vi "Read ini.vi"(8 "error in (no error)":errorcluster, 11 "Sett data":T1={"Filter"=0, "Gain"=0.0, "Bit rate"=0.0, "ISO/IEC w "=enum."14443 Type A", "BI"={"R"=0.0, "C"=0.0, "L"=0.0}, "BM"={"R"=0.0, "C"=0.0, "L"=0.0}, "M"={"Метка"=4, "Считыветель"=4}, "Type noise"=enum."Гауссовский шум", "Link"=enum."UPLINK", "Noise attenuator"=0.0, "Signal gain"=1.0, "Distance"=0.0} {"Distance" scale=0.0..10.0; "Signal gain" min=1.0 max=100.0 step=1.0 scale=1.0..30.0; "Noise attenuator" scale=0.01..1.01; "M"."Считыветель" min=4 max=128 step=4; "M"."Метка" min=4 max=128 step=4; "Bit rate" min=4.0 max=128.0 step=4.0}) -> (0 "error out":errorcluster, 3 "Sett data out":T1={"Filter"=0, "Gain"=0.0, "Bit rate"=0.0, "ISO/IEC w "=enum."14443 Type A", "BI"={"R"=0.0, "C"=0.0, "L"=0.0}, "BM"={"R"=0.0, "C"=0.0, "L"=0.0}, "M"={"Метка"=4, "Считыветель"=4}, "Type noise"=enum."Гауссовский шум", "Link"=enum."UPLINK", "Noise attenuator"=0.0, "Signal gain"=1.0, "Distance"=0.0} {"Distance" scale=0.0..10.0; "Signal gain" min=1.0 max=100.0 step=1.0 scale=1.0..30.0; "Noise attenuator" scale=0.01..1.01; "M"."Считыветель" min=4 max=128 step=4; "M"."Метка" min=4 max=128 step=4; "Bit rate" min=4.0 max=128.0 step=4.0})   [LabVIEW 2019]
uses:
  TypeDef/Sett data.ctl
  TypeDef/ISO.ctl
  TypeDef/Noise.ctl
  TypeDef/Link.ctl
  <vilib>/Utility/config.llb/Read Key (I32).vi
  <vilib>/Utility/config.llb/Read Key (Double).vi
  <vilib>/Utility/config.llb/NI_LVConfig.lvlib
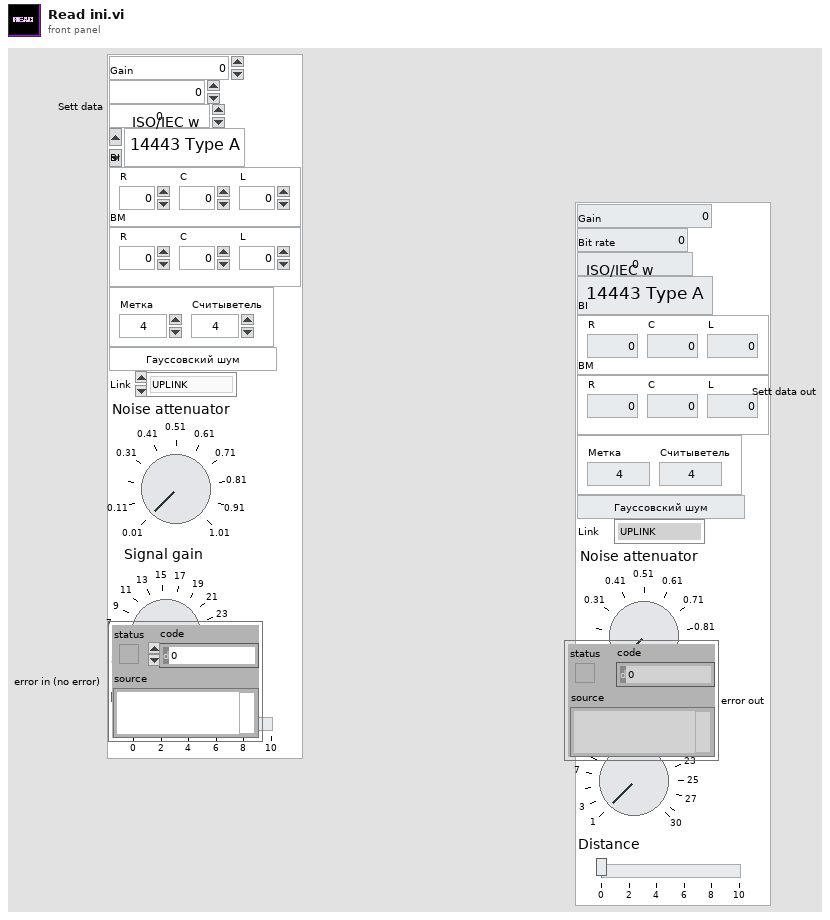
[diagram p1: front panel]
types:
  T1 = typedef "Sett data.ctl" = cluster{"Filter":i32, "Gain":dbl, "Bit rate":dbl, "ISO/IEC w ":T2, "BI":cluster{"R":dbl, "C":dbl, "L":dbl}, "BM":cluster{"R":dbl, "C":dbl, "L":dbl}, "M":cluster{"Метка":i64, "Считыветель":i64}, "Type noise":T3, "Link":T4, "Noise attenuator":dbl, "Signal gain":dbl, "Distance":dbl}
  T2 = typedef "ISO.ctl" = enum16{"14443 Type A", "14443 Type B", "Felica", "15693"}
  T3 = typedef "Noise.ctl" = enum16{"Гауссовский шум", "Белый шум"}
  T4 = typedef "Link.ctl" = enum16{"UPLINK", "DOWNLINK"}
  T5 = typedef "NI_LVConfig.lvlib/Config Data RefNum.ctl" = refnum<k1>
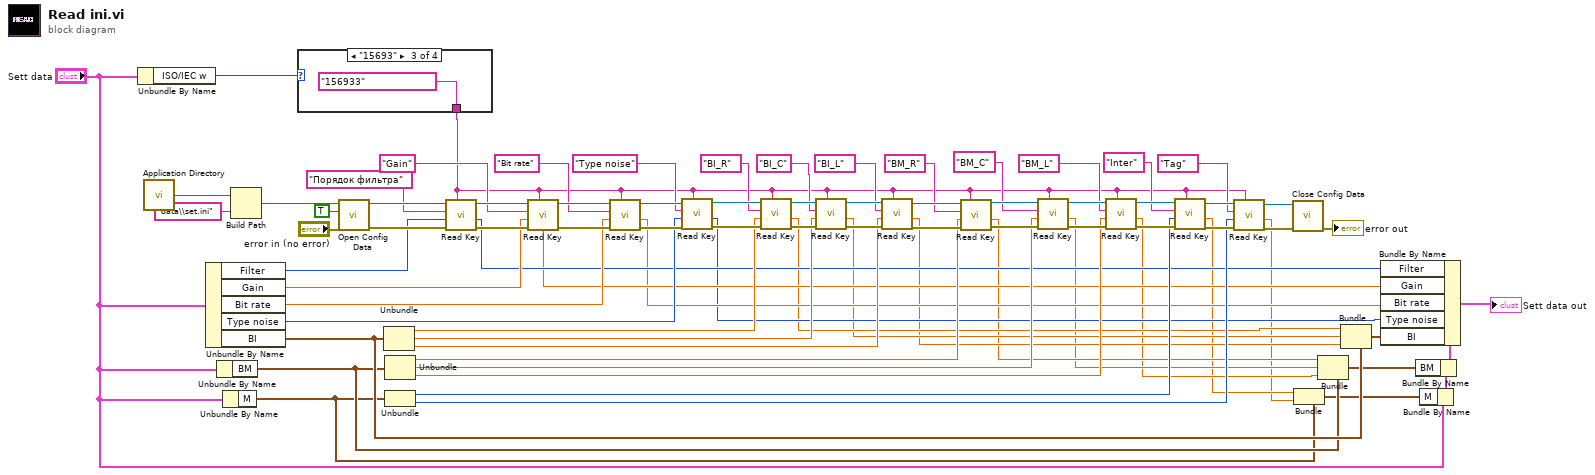
[diagram p0: block diagram]
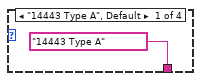
[diagram p2: hidden frame]
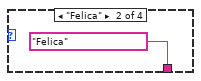
[diagram p3: hidden frame]
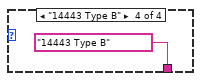
[diagram p4: hidden frame]
diagram:
  n1 = Unbundle By Name("Sett data") -> ("ISO/IEC w"=w73:T2)
  n2 = call <vilib>:"Application Directory.vi"() -> ("Application Directory"=w80:path)
  n3 = Unbundle By Name("Sett data") -> ("Filter"=w62:i32, "Gain"=w59:dbl, "Bit rate"=w58:dbl, "Type noise"=w56:T3, "BI"=w15:cluster{"R":dbl, "C":dbl, "L":dbl})
  n4 = Unbundle By Name("Sett data") -> ("BM"=w10:cluster{"R":dbl, "C":dbl, "L":dbl})
  n5 = Unbundle By Name("Sett data") -> ("M"=w4:cluster{"Метка":i64, "Считыветель":i64})
  n6 = Build Path(base path=w80, name or relative path="data\\set.ini") -> (appended path=w78:path)
  n7 = case shown="\"15693\"" w73 {
    tunnel: ["14443 Type A" "Felica" "156933" "14443 Type B"] -> w23
    frame "14443 Type A", Default {
    }
    frame "Felica" {
    }
    frame "15693" {
    }
    frame "14443 Type B" {
    }
  }
  n8 = call <vilib>:"Open Config Data.vi"("error in (no error)"="error in (no error)", "create file if necessary (T)"=TRUE, "configuration file path"=w78) -> ("error out"=w76:errorcluster, "refnum"=w72:T5)  [unwired: 6 in, 1 out]
  n9 = Unbundle(w15) -> ("R"=w36:dbl, "C"=w35:dbl, "L"=w34:dbl)
  n10 = Unbundle(w10) -> ("R"=w30:dbl, "C"=w29:dbl, "L"=w28:dbl)
  n11 = Unbundle(w4) -> ("Метка"=w27:i64, "Считыветель"=w26:i64)
  n12 = call-poly <vilib>:"Read Key.vi"("section"=w23, "error in (no error)"=w76, "default value"=w62, "key"="Порядок фильтра", "refnum"=w72) -> ("error out"=w75:errorcluster, "value"=w22:i32, "refnum out"=w71:T5)  [unwired: 3 in, 1 out]
  n13 = call-poly <vilib>:"Read Key.vi"("section"=w23, "error in (no error)"=w75, "default value"=w59, "key"="Gain", "refnum"=w71) -> ("error out"=w74:errorcluster, "value"=w21:dbl, "refnum out"=w70:T5)  [unwired: 3 in, 1 out]
  n14 = call-poly <vilib>:"Read Key.vi"("section"=w23, "error in (no error)"=w74, "default value"=w58, "key"="Bit rate", "refnum"=w70) -> ("error out"=w69:errorcluster, "value"=w20:dbl, "refnum out"=w66:T5)  [unwired: 3 in, 1 out]
  n15 = call-poly <vilib>:"Read Key.vi"("section"=w23, "error in (no error)"=w69, "default value"=w56, "key"="Type noise", "refnum"=w66) -> ("error out"=w68:errorcluster, "value"=w19:i32, "refnum out"=w67:T5)  [unwired: 3 in, 1 out]
  n16 = call-poly <vilib>:"Read Key.vi"("section"=w23, "error in (no error)"=w68, "default value"=w36, "key"="BI_R", "refnum"=w67) -> ("error out"=w42:errorcluster, "value"=w18:dbl, "refnum out"=w43:T5)  [unwired: 3 in, 1 out]
  n17 = call-poly <vilib>:"Read Key.vi"("section"=w23, "error in (no error)"=w42, "default value"=w35, "key"="BI_C", "refnum"=w43) -> ("error out"=w54:errorcluster, "value"=w17:dbl, "refnum out"=w55:T5)  [unwired: 3 in, 1 out]
  n18 = call-poly <vilib>:"Read Key.vi"("section"=w23, "error in (no error)"=w54, "default value"=w34, "key"="BI_L", "refnum"=w55) -> ("error out"=w52:errorcluster, "value"=w16:dbl, "refnum out"=w53:T5)  [unwired: 3 in, 1 out]
  n19 = call-poly <vilib>:"Read Key.vi"("section"=w23, "error in (no error)"=w52, "default value"=w30, "key"="BM_R", "refnum"=w53) -> ("error out"=w50:errorcluster, "value"=w9:dbl, "refnum out"=w51:T5)  [unwired: 3 in, 1 out]
  n20 = call-poly <vilib>:"Read Key.vi"("section"=w23, "error in (no error)"=w50, "default value"=w29, "key"="BM_C", "refnum"=w51) -> ("error out"=w48:errorcluster, "value"=w8:dbl, "refnum out"=w49:T5)  [unwired: 3 in, 1 out]
  n21 = call-poly <vilib>:"Read Key.vi"("section"=w23, "error in (no error)"=w48, "default value"=w28, "key"="BM_L", "refnum"=w49) -> ("error out"=w46:errorcluster, "value"=w7:dbl, "refnum out"=w47:T5)  [unwired: 3 in, 1 out]
  n22 = call-poly <vilib>:"Read Key.vi"("section"=w23, "error in (no error)"=w46, "default value"=w27, "key"="Inter", "refnum"=w47) -> ("error out"=w44:errorcluster, "value"=w3:dbl, "refnum out"=w45:T5)  [unwired: 3 in, 1 out]
  n23 = call-poly <vilib>:"Read Key.vi"("section"=w23, "error in (no error)"=w44, "default value"=w26, "key"="Tag", "refnum"=w45) -> ("error out"=w40:errorcluster, "value"=w2:dbl, "refnum out"=w41:T5)  [unwired: 3 in, 1 out]
  n24 = call <vilib>:"Close Config Data.vi"("error in (no error)"=w40, "refnum"=w41) -> ("error out"=→"error out":errorcluster)  [unwired: 8 in, 1 out]
  n25 = Bundle(cluster=w4, "Метка"=w3, "Считыветель"=w2) -> (w5:cluster{"Метка":i64, "Считыветель":i64})
  n26 = Bundle(cluster=w10, "R"=w9, "C"=w8, "L"=w7) -> (w6:cluster{"R":dbl, "C":dbl, "L":dbl})
  n27 = Bundle(cluster=w15, "R"=w18, "C"=w17, "L"=w16) -> (w14:cluster{"R":dbl, "C":dbl, "L":dbl})
  n28 = Bundle By Name(cluster="Sett data", "M"=w5) -> (w12:T1)
  n29 = Bundle By Name(cluster=w12, "BM"=w6) -> (w11:T1)
  n30 = Bundle By Name(cluster=w11, "Filter"=w22, "Gain"=w21, "Bit rate"=w20, "Type noise"=w19, "BI"=w14) -> (→"Sett data out":T1)
